vi "PicoScope6000GetValuesOverlappedBulk.vi"(5 "Segment Range":T1 {"toSegmentIndex" format="%.4p"; "fromSegmentIndex" format="%.4p"}, 7 "Buffer and Transfer Settings":T2 {"Down-Sample Mode" items=["RAW none", "None", "Aggregate", "Decimate", "Average"]; "Down Sample Ratio" step=1; "Samples" format="%_6p"}, 8 "error in (no error)":errorcluster, 11 "handle in":i16) -> (0 "error out":errorcluster, 3 "handle out":i16, 4 "overflow":u64[](array[numeric]) format="%010b", 6 "noOfSamples":u64)   [LabVIEW 2009]
doc: "Calls ps5000aGetValuesOverlapped"
uses:
  ps6000.dll
  shared/Segment Range.ctl
  shared/Buffer and Transfer Settings.ctl
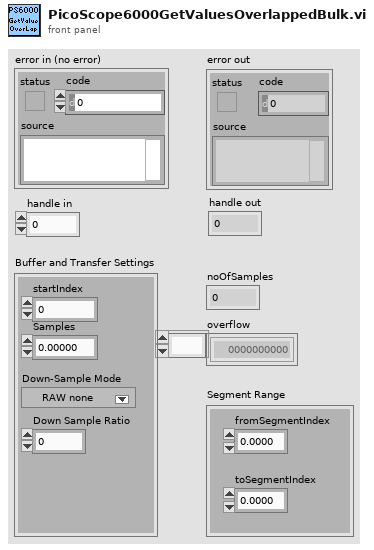
[diagram p1: front panel]
types:
  T1 = typedef "Segment Range.ctl" = cluster{"fromSegmentIndex":u64, "toSegmentIndex":u64}
  T2 = typedef "Buffer and Transfer Settings.ctl" = cluster{"startIndex":u64, "Samples":u64, "Down Sample Ratio":u64, "Down-Sample Mode":u32}
  T3 = cluster{"status":bool, "code":u32, "source":string}
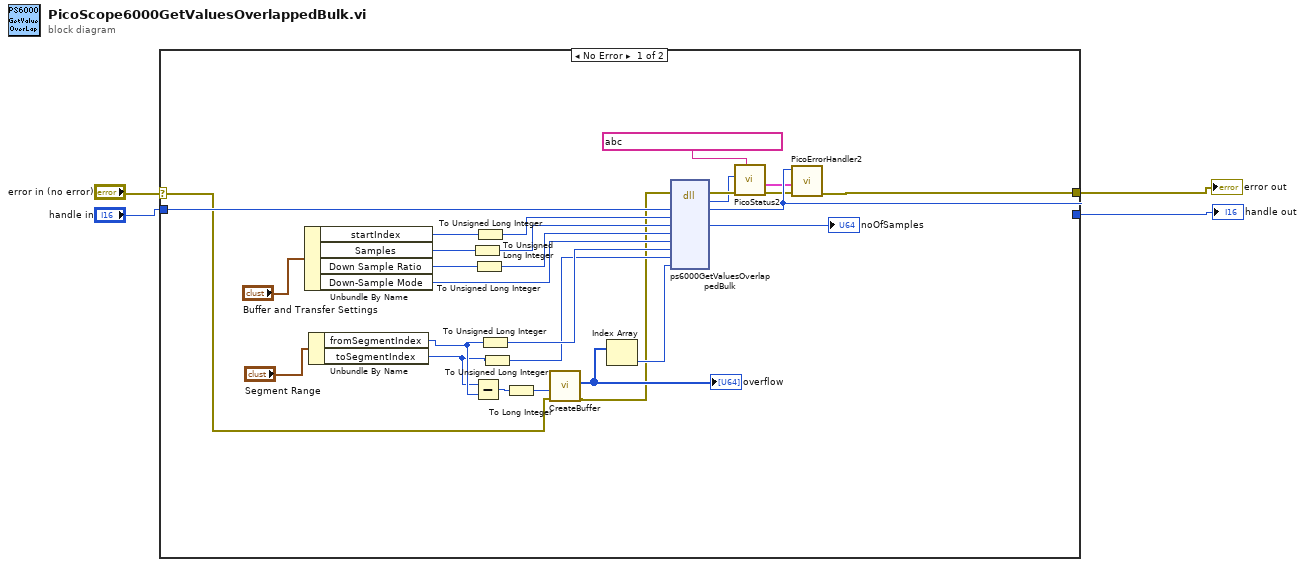
[diagram p0: block diagram]
diagram:
  n1 = case shown="No Error" "error in (no error)" {
    selector: "error in (no error)" -> [w6 w33]
    tunnel: "handle in" -> [w30 w34]
    tunnel: [w28 w34] -> w4
    tunnel: [w29 w33] -> w3
    frame #0 {
      n2 = Unbundle By Name("Buffer and Transfer Settings") -> ("startIndex"=w20:u64, "Samples"=w18:u64, "Down Sample Ratio"=w16:u64, "Down-Sample Mode"=w32:u32)
      n3 = Unbundle By Name("Segment Range") -> ("fromSegmentIndex"=w12:u64, "toSegmentIndex"=w11:u64)
      n4 = To Unsigned Long Integer(number=w18) -> (unsigned 32bit integer=w17:u32)
      n5 = Subtract(x=w11, y=w12) -> (x-y=w14:u64)
      n6 = To Unsigned Long Integer(number=w16) -> (unsigned 32bit integer=w15:u32)
      n7 = To Unsigned Long Integer(number=w20) -> (unsigned 32bit integer=w19:u32)
      n8 = To Unsigned Long Integer(number=w12) -> (unsigned 32bit integer=w10:u32)
      n9 = To Unsigned Long Integer(number=w11) -> (unsigned 32bit integer=w9:u32)
      n10 = To Long Integer(number=w14) -> (32bit integer=w13:i32)
      n11 = call "CreateBuffer.vi"("error in (no error)"=w6, "Buffer size"=w13) -> ("error out"=w5:errorcluster, "Pointer and BufferSize"=w7:u64[])  [unwired: 8 in]
      "overflow" <- w7
      n12 = Index Array(array=w7) -> (element=w8:u64)  [unwired: 1 in]
      n13 = dll-call lib="ps6000.dll" fn="ps6000GetValuesOverlappedBulk" ("ps3000.dll:_ps3000_open_unit@0")(error in=w5, "handle"=w30, "startIndex"=w19, "noOfSamples"=w17, "downSampleRatio"=w15, "downSampleRatioMode"=w32, "fromSegmentIndex"=w10, "toSegmentIndex"=w9, "overflow"=w8) -> (error out=w24:errorcluster, "PICO_STATUS"=w21:u32, "handle"=w28:i16, "noOfSamples"=→"noOfSamples":u32)  [unwired: 8 in, 1 out]
      n14 = call "PicoStatus2.vi"("PICO source"=string ? ("source"), "Error in"=w24, "PICO STATUS"=w21) -> ("error out"=w25:errorcluster, "PICO_STATUS out"=w22:T3)  [unwired: 5 in]
      n15 = call "PicoErrorHandler2.vi"("error in (no error)"=w25, "PICO_STATUS in"=w22, "handle In"=w28) -> ("error out"=w29:errorcluster)  [unwired: 8 in]
    }
    frame #1 {
    }
  }
  "error out" <- w3
  "handle out" <- w4
